vi "SDA - Analise e calibracao - backup 04.12.18.vi"() -> ()   [LabVIEW 2014]
uses:
  <vilib>/Utility/file.llb/Read From Spreadsheet File (DBL).vi
  <vilib>/Analysis/NI_AALPro.lvlib
  <vilib>/gmath/NI_Gmath.lvlib
  <vilib>/measure/NI_MABase.lvlib
panel:
  in  "Amplitude base":dbl=1.25 format="%#_13g"
  in  "p.u. ?":bool=TRUE
  in  "Numeric":dbl
  out "output cluster":cluster{i32, i32}
  in  "offset":dbl format="%0.2p"
  in  "phase":dbl format="%.2p"
  in  "amplitude":dbl=1.0 format="%0.2p"
  in  "frequency":dbl=10.0 format="%0.2p"
  out "delay time":dbl format="%#_6f"
  in  "y":dbl
  out "fractional index or x":dbl format="%#_7g"
  in  "threshold y":dbl=0.95
  out "spread value":dbl
  out "lenght":i32
  in  "kept interval":i32=25
  out "Table 2":string[][](table)
  in  "Labels Size":u32=24
  in  "X label":T1(ring)=enum."medidas"
  in  "Tab Control":T2(tab)
  in  "Tab Control 2":T3(tab)
  out "Magnitude absolute deviation":dbl[](graph)
  out "Absolute phase deviation":dbl[](graph)
  out "Magnitude deviation":dbl[](graph)
  out "Phase deviation":dbl[](graph)
  out "Phase":dbl[][](graph)
  out "Magnitude":dbl[][](graph)
  out "TVE":dbl[](graph)
  in  "Tab Control 3":T3(tab)
  out "Absolute freq. deviation":dbl[](graph)
  out "Absolute ROCOF deviation":dbl[](graph)
  out "Frequency deviation":dbl[](graph)
  out "ROCOF deviation":dbl[](graph)
  out "Frequency":dbl[][](graph)
  out "ROCOF":dbl[][](graph)
  out "Curve fit":dbl[][](graph)
  out "ROCOF\nreference":dbl[](array[numeric])
  out "ROCOF\nmeasured":dbl[](array[numeric])
  out "Frequency\nmeasured":dbl[](array[numeric])
  out "Frequency\nreference":dbl[](array[numeric])
  out "Phase\nmeasured":dbl[](array[numeric])
  out "Phase\nreference":dbl[](array[numeric])
  out "Magnitude\nmeasured":dbl[](array[numeric])
  out "Magnitude\nreference":dbl[](array[numeric])
  in  "polynomial order":i32=2
  in  "Type":T4(ring)=enum."Linear"
  out "Coefficients":string[][](table) caption="Table"
  in  "X data":T5(ring)
  in  "Y data":T5(ring)=enum."Magnitude deviation"
  out "Fit deviation":dbl[](graph)
  out "Correlation\ncoefficient (R)":dbl format="%.7g"
  out "R^2":dbl format="%.7g"
  in  "busca freq":dbl
  out "XY Graph 3":cluster{dbl[], dbl[]}(graph)
  out "XY Graph 2":cluster{dbl[], dbl[]}(graph)
  out "fractional index":dbl format="%_6g"
  out "x*y":dbl
  in  "fractional index or x 3":dbl
  out "ângulo corresp":dbl
  out "mag correspondente":dbl
  in  "frequency 2":dbl
  out "TVE Histogram":T6(graph)
  out "Frequency Error Histogram":T6(graph)
  out "Magnitude Error Histogram":T6(graph)
  out "Phase Error Histogram":T6(graph)
  in  "final":i32
  in  "Interval":bool
  in  "index":i32
  out "nº de amostras":i32
  in  "del interval":i32=25
  in  "Exclude\ninterval":bool
  in  "Archive name":path=path "D:/Resultados/teste.txt"
  # "Fase x freq"
  # "Mag. x mag."
  # "Synchrophasors Data Analysis"
  # "Main Errors"
  # "Max"
  # "Mean"
  # "Min"
  # "Magnitude (%)"
  # "Phase (º)"
  # "TVE (%)"
  # "Freq. (Hz)"
  # "ROCOF (Hz/s)"
  # "Tamanho para dissertação:\n312x732"
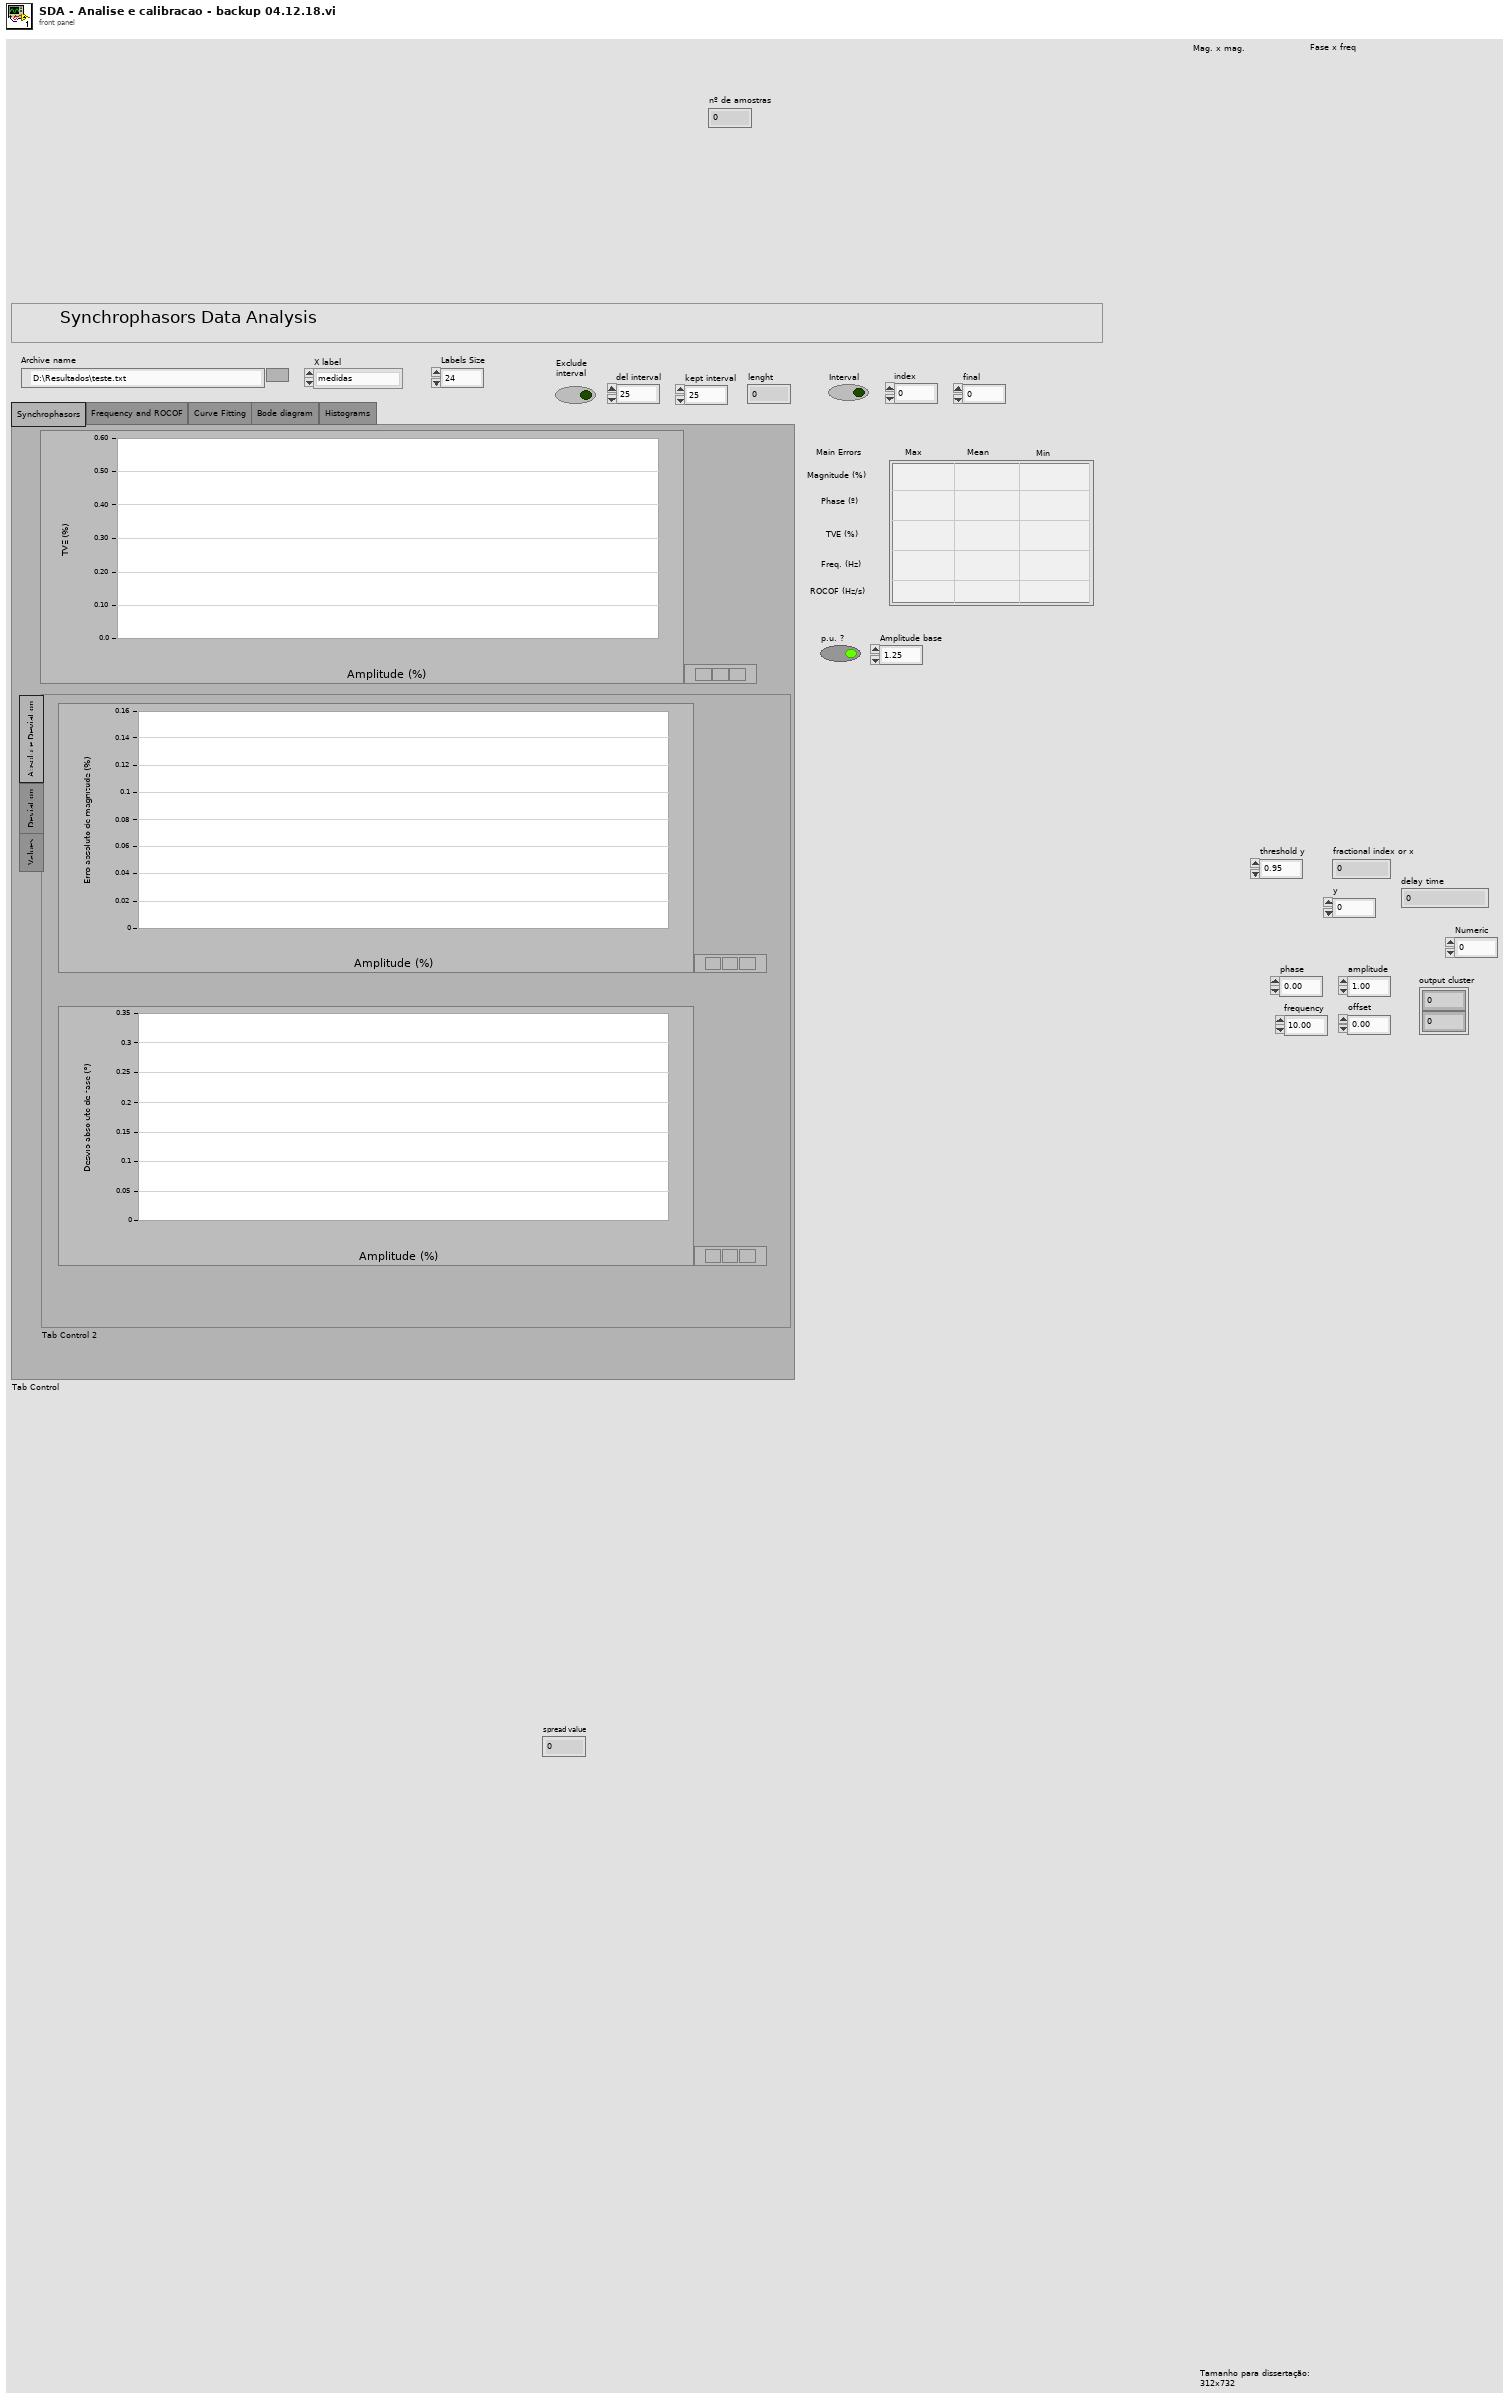
[diagram p1: front panel]
types:
  T1 = enum16{"tempo (s)", "medidas", "Amplitude (%)", "Ângulo (°)", "Frequência (Hz)", "ROCOF (Hz/s)", "Harmônica (.ª)", "Frequência de interferência (Hz)", "Frequência de modulação (Hz)"}
  T2 = enum32{"Synchrophasors", "Frequency and ROCOF", "Curve Fitting", "Bode diagram", "Histograms"}
  T3 = enum32{"Absolute Deviation", "Deviation", "Values"}
  T4 = enum16{"Exponencial", "Logarithm", "Linear", "Polynomial", "Sinusoidal"}
  T5 = enum16{"Magnitude reference", "Magnitude measured", "Magnitude deviation", "Phase reference", "Phase measured", "Phase deviation", "Frequency reference", "Frequency measured", "Frequency deviation"}
  T6 = cluster{"X Values":dbl[], "Histogram: h(x)":i32[]}
  T7 = cluster{"max ref":dbl, "min ref":dbl, "mean ref":dbl, "max dev":dbl, "min dev":dbl, "mean dev":dbl, "max meas":dbl, "min meas":dbl, "mean meas":dbl}
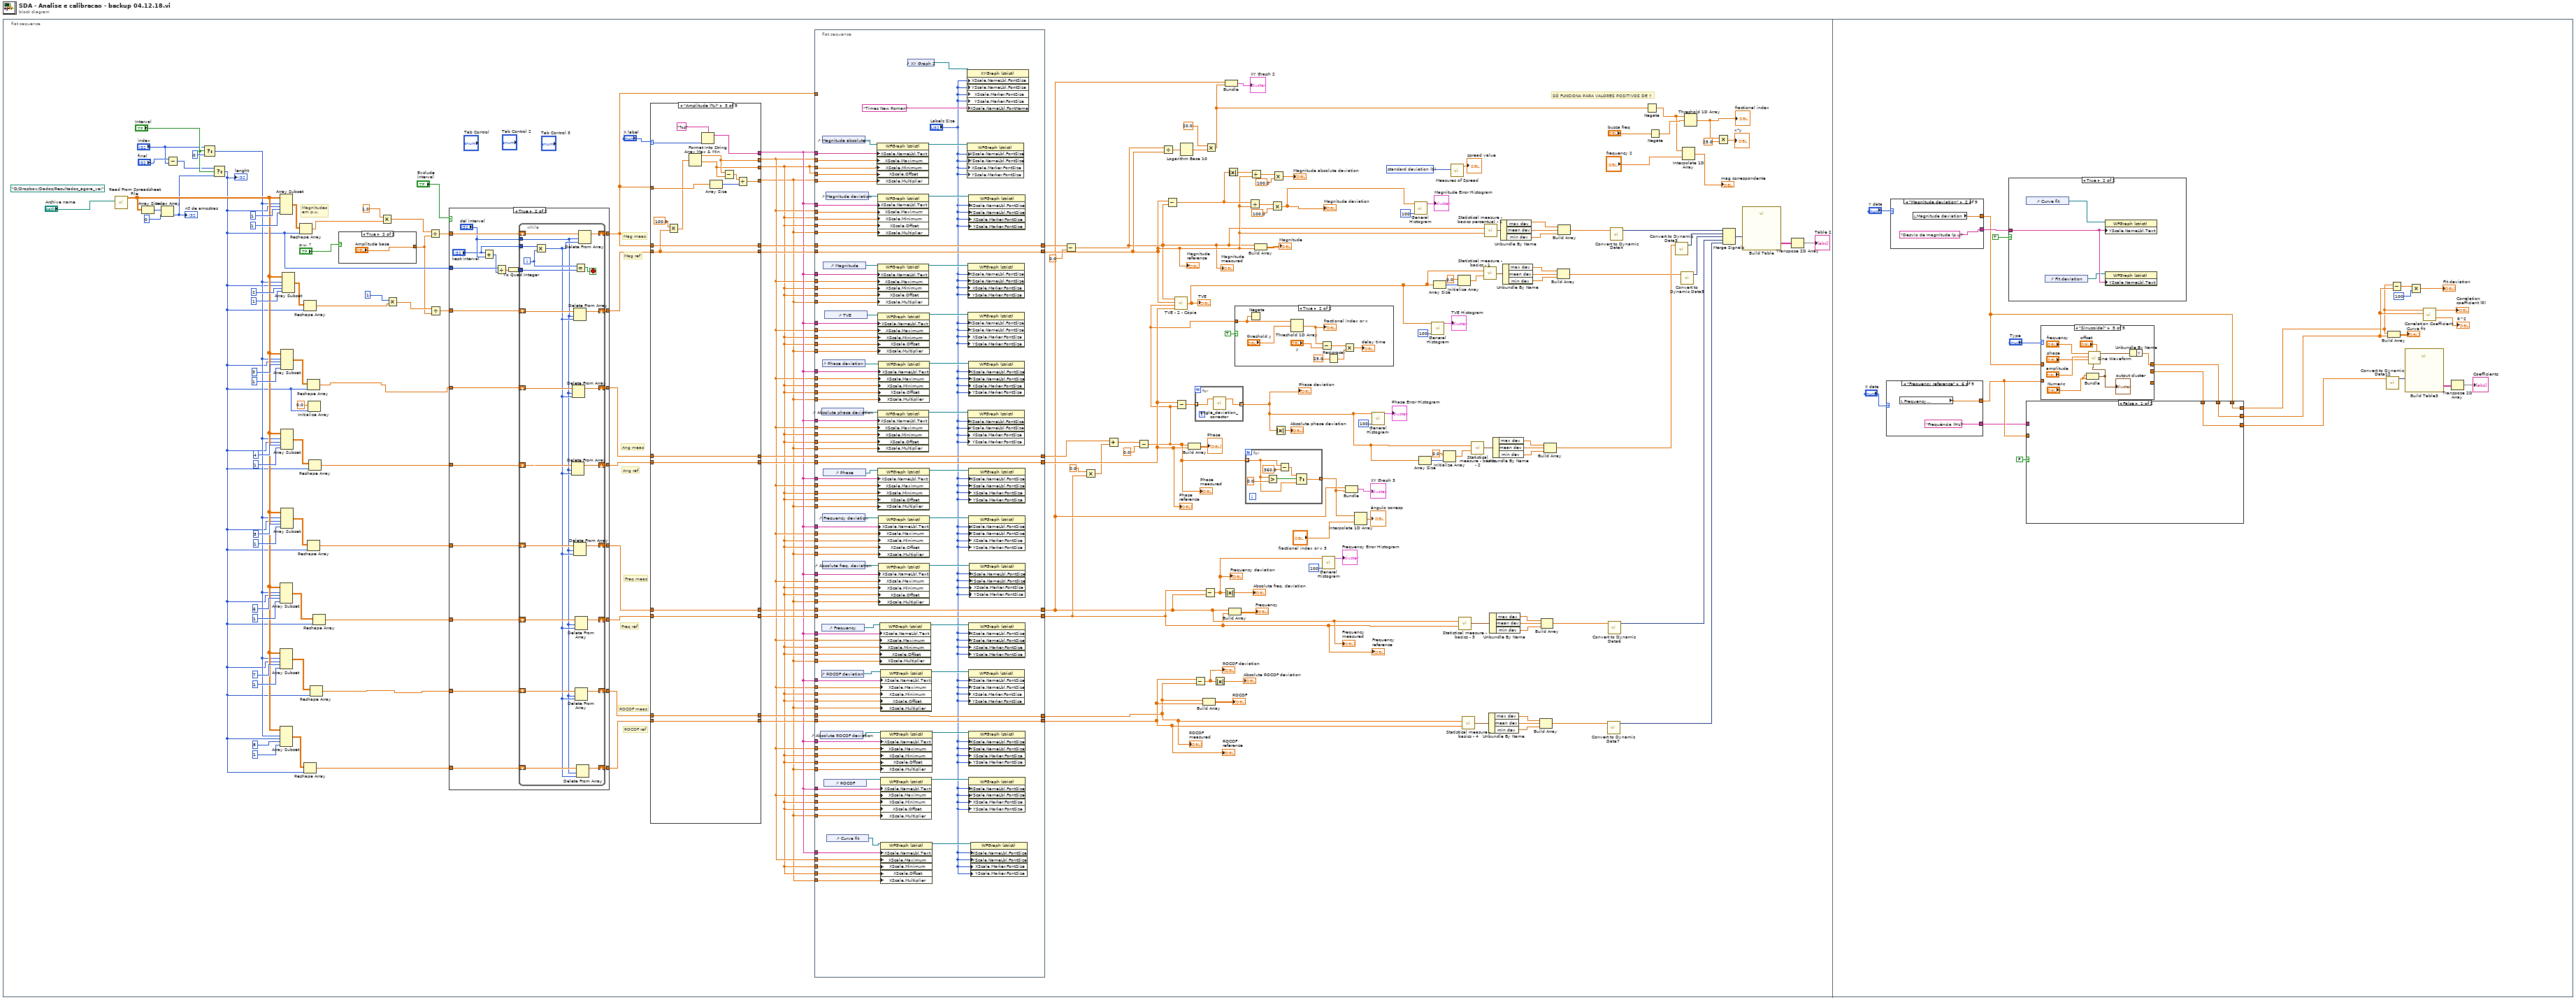
[diagram p0: block diagram]
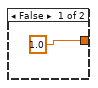
[diagram p3: hidden frame]
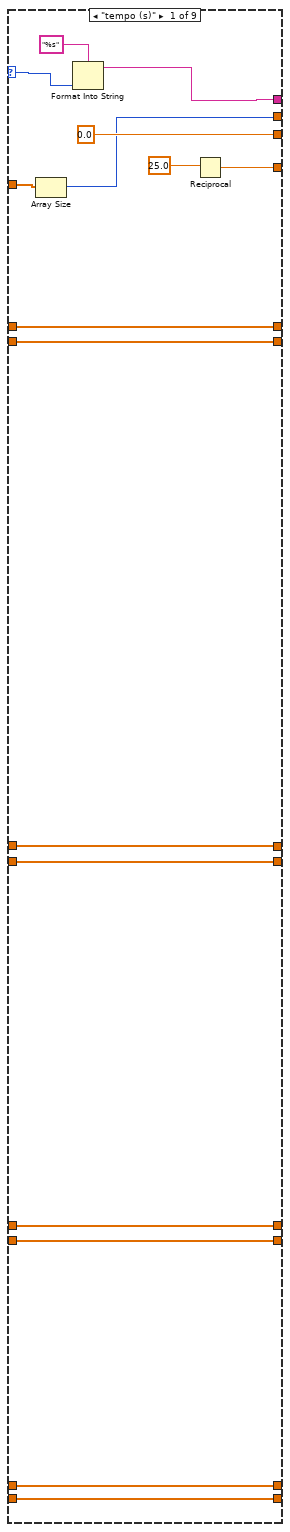
[diagram p4: hidden frame]
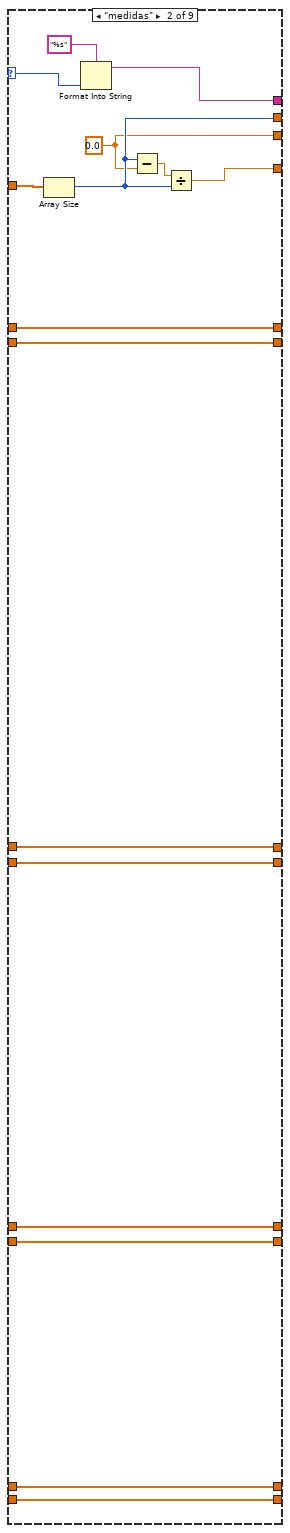
[diagram p5: hidden frame]
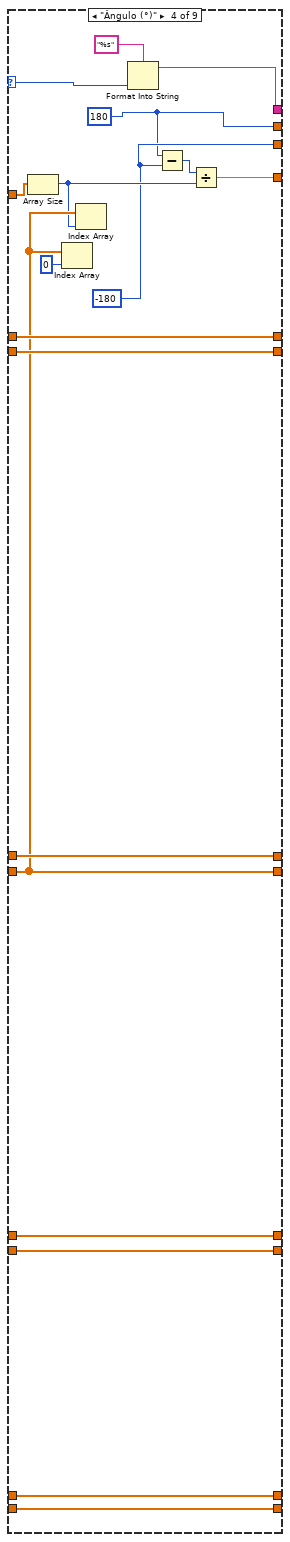
[diagram p6: hidden frame]
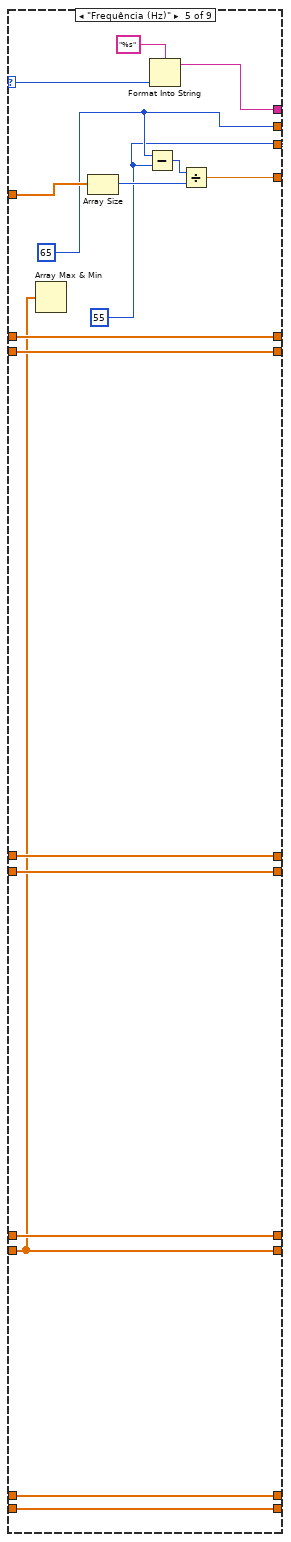
[diagram p7: hidden frame]
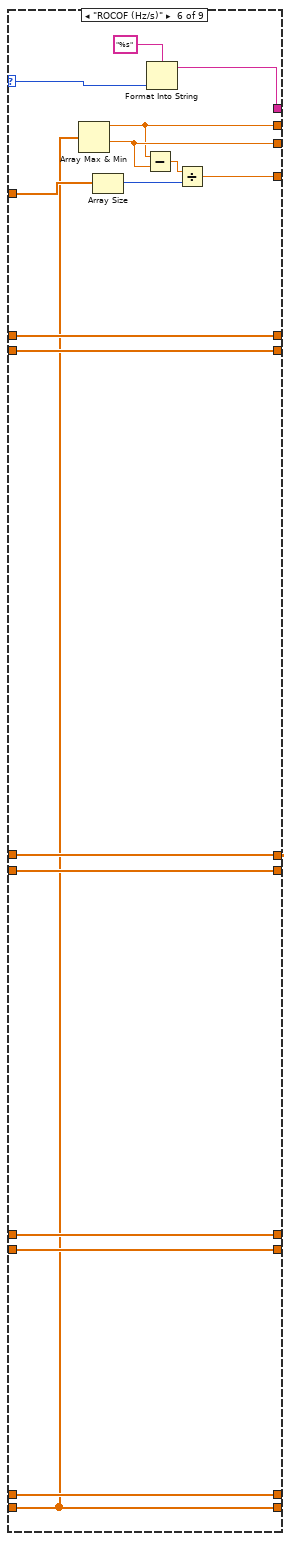
[diagram p8: hidden frame]
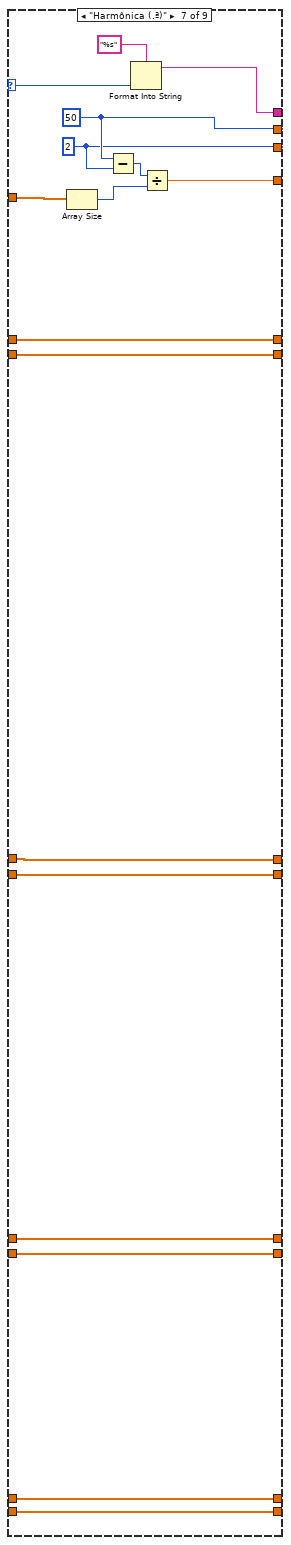
[diagram p9: hidden frame]
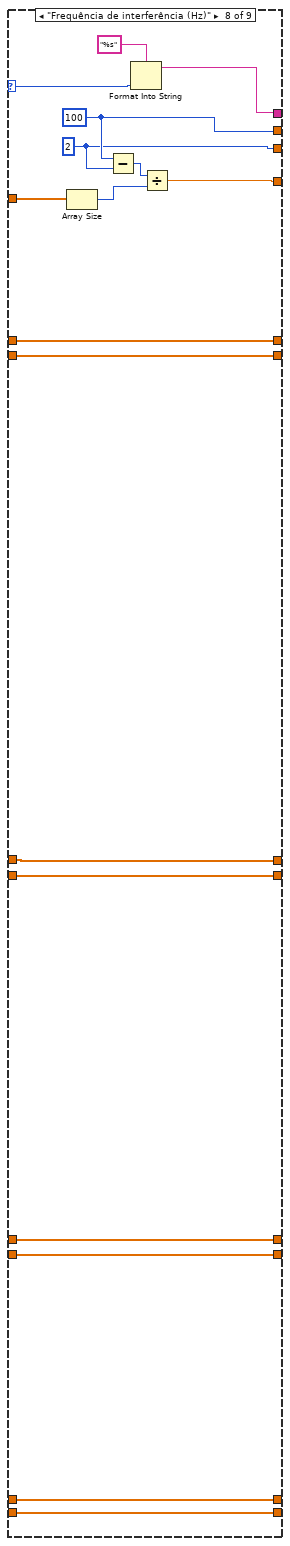
[diagram p10: hidden frame]
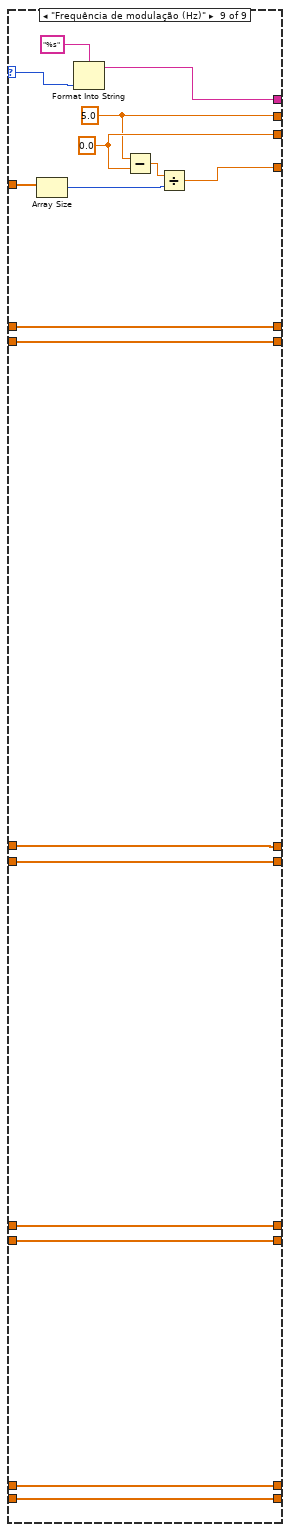
[diagram p11: hidden frame]
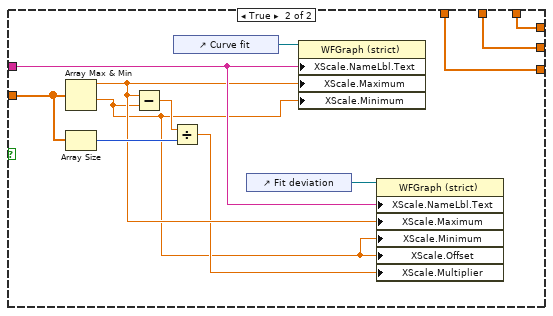
[diagram p13: hidden frame]
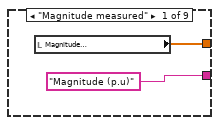
[diagram p15: hidden frame]
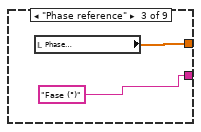
[diagram p16: hidden frame]
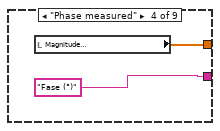
[diagram p17: hidden frame]
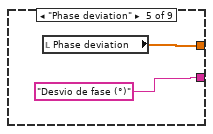
[diagram p18: hidden frame]
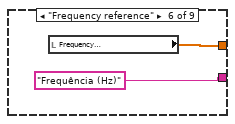
[diagram p19: hidden frame]
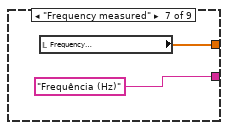
[diagram p20: hidden frame]
diagram:
  n1 = flat-sequence {
    frame #0 {
      w60 = 0 items=["standard deviation", "range", "mean absolute deviation", "interquartile range"] ("type")
      (unwired) path "D:/Dropbox/Dados/Resultados_agora_vai" ("file path (use dialog)")
      # "SÓ FUNCIONA PARA VALORES POSITIVOS DE Y"
      # "Magnitudes\nem p.u."
      # "ROCOF ref"
      # "ROCOF meas"
      # "Freq ref"
      # "Freq meas"
      # "Ang ref"
      # "Ang meas"
      # "Mag meas"
      # "Mag ref"
      n2 = call-poly <vilib>:"Read From Spreadsheet File.vi"("file path (dialog if empty)"="Archive name") -> ("all rows"=w151:dbl[][])  [unwired: 6 in, 4 out]
      n3 = Array Size(array=w151) -> (size(s)=w174:i32[])
      n4 = Index Array(array=w174, index=0) -> (element=w104:i32)
      "nº de amostras" <- w104
      n5 = Subtract(x="final", y="index") -> (x-y=w107:i32)
      n6 = Select(t="index", s="Interval", f=0) -> (s? t:f=w124:i32)
      n7 = Select(t=w107, s="Interval", f=w104) -> (s? t:f=w22:i32)
      "lenght" <- w22
      n8 = Array Subset(array=w151, index (row)=w124, length (row)=w22, index (col)=1 ("index"), length (col)=1 ("length")) -> (w175:dbl[][])
      n9 = Array Subset(array=w151, index (row)=w124, length (row)=w22, index (col)=6 ("index"), length (col)=1 ("length")) -> (w158:dbl[][])
      n10 = Array Subset(array=w151, index (row)=w124, length (row)=w22, index (col)=7 ("index"), length (col)=1 ("length")) -> (w155:dbl[][])
      n11 = Array Subset(array=w151, index (row)=w124, length (row)=w22, index (col)=8 ("index"), length (col)=1 ("length")) -> (w74:dbl[][])
      n12 = Array Subset(array=w151, index (row)=w124, length (row)=w22, index (col)=4 ("index"), length (col)=1 ("length")) -> (w164:dbl[][])
      n13 = Array Subset(array=w151, index (row)=w124, length (row)=w22, index (col)=5 ("index"), length (col)=1 ("length")) -> (w161:dbl[][])
      n14 = Array Subset(array=w151, index (row)=w124, length (row)=w22, index (col)=3 ("index"), length (col)=1 ("length")) -> (w167:dbl[][])
      n15 = Array Subset(array=w151, index (row)=w124, length (row)=w22, index (col)=2 ("index"), length (col)=1 ("length")) -> (w170:dbl[][])
      n16 = Reshape Array(w175, w22) -> (w52:dbl[])
      n17 = Reshape Array(w170, w22) -> (w50:dbl[])
      n18 = Reshape Array(w74, w22) -> (w73:dbl[])
      n19 = Reshape Array(w167, w22) -> (w21:dbl[])
      n20 = Reshape Array(w161, w22) -> (w126:dbl[])
      n21 = Initialize Array(0.0 ("element"), w22) -> ()  [unwired: 1 out]
      n22 = Reshape Array(w164, w22) -> (w125:dbl[])
      n23 = Reshape Array(w155, w22) -> (w4:dbl[])
      n24 = Reshape Array(w158, w22) -> (w127:dbl[])
      n25 = case shown="True" "p.u. ?" {
        tunnel: [1.0 "Amplitude base"] -> w3
        frame False {
        }
        frame True {
        }
      }
      n26 = Multiply(x=1.0, y=w52) -> (x*y=w51:dbl[])
      n27 = Multiply(x=1, y=w50) -> (x*y=w49:dbl[])
      n28 = Divide(x=w51, y=w3) -> (x/y=w84:dbl[])
      n29 = Divide(x=w49, y=w3) -> (x/y=w83:dbl[])
      n30 = case shown="True" "Exclude\ninterval" {
        tunnel: w84 -> [w466 w488]
        tunnel: [w466 w487] -> w41
        tunnel: w73 -> [w459 w483]
        tunnel: w4 -> [w460 w469]
        tunnel: w127 -> [w461 w480]
        tunnel: w126 -> [w462 w478]
        tunnel: w125 -> [w463 w476]
        tunnel: w21 -> [w464 w484]
        tunnel: w83 -> [w465 w486]
        tunnel: [w465 w485] -> w102
        tunnel: [w464 w474] -> w100
        tunnel: [w463 w475] -> w101
        tunnel: [w462 w477] -> w99
        tunnel: [w461 w479] -> w98
        tunnel: [w460 w481] -> w96
        tunnel: [w459 w482] -> w97
        tunnel: w22 -> [_ w473]
        frame False {
        }
        frame True {
          n31 = Add(x="kept interval", y="del interval") -> (x+y=w471:i32)
          n32 = Divide(x=w473, y=w471) -> (x/y=w468:dbl)
          n33 = To Quad Integer(1:w468) -> (0:w467:i64)
          n34 = while {
            tunnel: "del interval" -> [w490]
            shift-right: [w508] -> w487
            shift-left: w488 -> [w509]
            shift-right: [w507] -> w485
            shift-left: w486 -> [w506]
            shift-right: [w504] -> w474
            shift-left: w484 -> [w505]
            shift-right: [w502] -> w475
            shift-left: w476 -> [w503]
            shift-right: [w500] -> w477
            shift-left: w478 -> [w501]
            shift-right: [w498] -> w479
            shift-left: w480 -> [w499]
            shift-right: [w496] -> w481
            shift-left: w469 -> [w497]
            shift-right: [w494] -> w482
            shift-left: w483 -> [w495]
            tunnel: w467 -> [w493]
            tunnel: "kept interval" -> [w489]
            i -> [w492]
            stop <- w510 stop-if-true
            n35 = Multiply(x=w489, y=w492) -> (x*y=w491:i32)
            n36 = Delete From Array(array=w503, length=w490, index=w491) -> (array with subset deleted=w502:dbl[])  [unwired: 1 out]
            n37 = Delete From Array(array=w505, length=w490, index=w491) -> (array with subset deleted=w504:dbl[])  [unwired: 1 out]
            n38 = Delete From Array(array=w506, length=w490, index=w491) -> (array with subset deleted=w507:dbl[])  [unwired: 1 out]
            n39 = Delete From Array(array=w501, length=w490, index=w491) -> (array with subset deleted=w500:dbl[])  [unwired: 1 out]
            n40 = Equal?(x=w492, y=w493) -> (x = y?=w510:bool)
            n41 = Delete From Array(array=w499, length=w490, index=w491) -> (array with subset deleted=w498:dbl[])  [unwired: 1 out]
            n42 = Delete From Array(array=w497, length=w490, index=w491) -> (array with subset deleted=w496:dbl[])  [unwired: 1 out]
            n43 = Delete From Array(array=w495, length=w490, index=w491) -> (array with subset deleted=w494:dbl[])  [unwired: 1 out]
            n44 = Delete From Array(array=w509, length=w490, index=w491) -> (array with subset deleted=w508:dbl[])  [unwired: 1 out]
          }
        }
      }
      n45 = case shown="\"Amplitude (%)\"" "X label" {
        selector: "X label" -> [w310 w325 w344 w364 w380 w398 w423 w432 w451]
        tunnel: w41 -> [w311 w326 w355 w363 w381 w399 w420 w429 w452]
        tunnel: w102 -> [w319 w335 w341 w372 w378 w396 w417 w440 w454]
        tunnel: [w319 w335 w341 w372 w378 w396 w417 w440 w454] -> w86
        tunnel: w41 -> [w320 w336 w352 w373 w390 w397 w418 w441 w455]
        tunnel: [w320 w336 w352 w373 w390 w397 w418 w441 w455] -> w85
        tunnel: w101 -> [w317 w333 w350 w360 w388 w406 w416 w439 w446]
        tunnel: w100 -> [w318 w334 w351 w371 w389 w407 w408 w425 w447]
        tunnel: [w318 w334 w351 w371 w389 w407 w408 w425 w447] -> w87
        tunnel: [w317 w333 w350 w360 w388 w406 w416 w439 w446] -> w88
        tunnel: w99 -> [w316 w332 w349 w370 w387 w405 w415 w438 w445]
        tunnel: w98 -> [w315 w331 w348 w369 w377 w404 w414 w437 w444]
        tunnel: [w316 w332 w349 w370 w387 w405 w415 w438 w445] -> w90
        tunnel: [w315 w331 w348 w369 w377 w404 w414 w437 w444] -> w89
        tunnel: w97 -> [w313 w329 w347 w367 w385 w393 w412 w435 w442]
        tunnel: [w313 w329 w347 w367 w385 w393 w412 w435 w442] -> w92
        tunnel: w96 -> [w314 w330 w346 w368 w386 w403 w413 w436 w443]
        tunnel: [w314 w330 w346 w368 w386 w403 w413 w436 w443] -> w91
        tunnel: [w309 w324 w343 w362 w379 w395 w419 w433 w456] -> w57
        tunnel: [w307 w323 w339 w356 w375 w392 w411 w428 w448] -> w56
        tunnel: [0.0 ("X Scale.Offset and Multiplier:Offset") w322 w338 w357 w374 w394 w410 w427 w449] -> w55
        tunnel: [w305 w321 w337 w358 w376 w391 w409 w426 w453] -> w54
        frame "tempo (s)" {
          n46 = Array Size(array=w311) -> (size(s)=w307:i32)
          n47 = Format Into String(format string="%s", w310) -> (resulting string=w309:string)  [unwired: 2 in, 1 out]
          n48 = Reciprocal(x=25.0 ("X Scale.Offset and Multiplier:Offset")) -> (1/x=w305:dbl)
        }
        frame "medidas" {
          w322 = 0.0 ("X Scale.Offset and Multiplier:Offset")
          n49 = Array Size(array=w326) -> (size(s)=w323:i32)
          n50 = Format Into String(format string="%s", w325) -> (resulting string=w324:string)  [unwired: 2 in, 1 out]
          n51 = Subtract(x=w323, y=w322) -> (x-y=w328:dbl)
          n52 = Divide(x=w328, y=w323) -> (x/y=w321:dbl)
        }
        frame "Amplitude (%)" {
          n53 = Multiply(x=100.0 ("y"), y=w341) -> (x*y=w340:dbl[])
          n54 = Array Max & Min(array=w340) -> (max value=w339:dbl, min value=w338:dbl)  [unwired: 2 out]
          n55 = Format Into String(format string="%s", w344) -> (resulting string=w343:string)  [unwired: 2 in, 1 out]
          n56 = Array Size(array=w355) -> (size(s)=w354:i32)
          n57 = Subtract(x=w339, y=w338) -> (x-y=w353:dbl)
          n58 = Divide(x=w353, y=w354) -> (x/y=w337:dbl)
        }
        frame "Ângulo (°)" {
          w356 = 180
          w357 = -180
          n59 = Array Size(array=w363) -> (size(s)=w359:i32)
          n60 = Index Array(array=w360, index=0) -> ()  [unwired: 1 out]
          n61 = Index Array(array=w360, index=w359) -> ()  [unwired: 1 out]
          n62 = Format Into String(format string="%s", w364) -> (resulting string=w362:string)  [unwired: 2 in, 1 out]
          n63 = Subtract(x=w356, y=w357) -> (x-y=w366:i32)
          n64 = Divide(x=w366, y=w359) -> (x/y=w358:dbl)
        }
        frame "Frequência (Hz)" {
          w374 = 55
          w375 = 65
          n65 = Array Max & Min(array=w377) -> ()  [unwired: 4 out]
          n66 = Array Size(array=w381) -> (size(s)=w384:i32)
          n67 = Subtract(x=w375, y=w374) -> (x-y=w383:i32)
          n68 = Format Into String(format string="%s", w380) -> (resulting string=w379:string)  [unwired: 2 in, 1 out]
          n69 = Divide(x=w383, y=w384) -> (x/y=w376:dbl)
        }
        frame "ROCOF (Hz/s)" {
          n70 = Array Max & Min(array=w393) -> (max value=w392:dbl, min value=w394:dbl)  [unwired: 2 out]
          n71 = Array Size(array=w399) -> (size(s)=w402:i32)
          n72 = Subtract(x=w392, y=w394) -> (x-y=w401:dbl)
          n73 = Format Into String(format string="%s", w398) -> (resulting string=w395:string)  [unwired: 2 in, 1 out]
          n74 = Divide(x=w401, y=w402) -> (x/y=w391:dbl)
        }
        frame "Harmônica (.ª)" {
          w410 = 2
          w411 = 50
          n75 = Array Size(array=w420) -> (size(s)=w422:i32)
          n76 = Subtract(x=w411, y=w410) -> (x-y=w421:i32)
          n77 = Format Into String(format string="%s", w423) -> (resulting string=w419:string)  [unwired: 2 in, 1 out]
          n78 = Divide(x=w421, y=w422) -> (x/y=w409:dbl)
        }
        frame "Frequência de interferência (Hz)" {
          w427 = 2
          w428 = 100
          n79 = Array Size(array=w429) -> (size(s)=w431:i32)
          n80 = Subtract(x=w428, y=w427) -> (x-y=w430:i32)
          n81 = Format Into String(format string="%s", w432) -> (resulting string=w433:string)  [unwired: 2 in, 1 out]
          n82 = Divide(x=w430, y=w431) -> (x/y=w426:dbl)
        }
        frame "Frequência de modulação (Hz)" {
          w448 = 5.0 ("X Scale.Offset and Multiplier:Offset")
          w449 = 0.0 ("X Scale.Offset and Multiplier:Offset")
          n83 = Array Size(array=w452) -> (size(s)=w450:i32)
          n84 = Format Into String(format string="%s", w451) -> (resulting string=w456:string)  [unwired: 2 in, 1 out]
          n85 = Subtract(x=w448, y=w449) -> (x-y=w458:dbl)
          n86 = Divide(x=w458, y=w450) -> (x/y=w453:dbl)
        }
      }
      n87 = flat-sequence {
        tunnel: w57 -> [w304]
        tunnel: w57 -> [w303]
        tunnel: w57 -> [w302]
        tunnel: w56 -> [w301]
        tunnel: w55 -> [w300]
        tunnel: w55 -> [w299]
        tunnel: w54 -> [w298]
        tunnel: w56 -> [w297]
        tunnel: w55 -> [w296]
        tunnel: w55 -> [w295]
        tunnel: w54 -> [w294]
        tunnel: w57 -> [w293]
        tunnel: w57 -> [w292]
        tunnel: w57 -> [w291]
        tunnel: w54 -> [w290]
        tunnel: w55 -> [w289]
        tunnel: w55 -> [w288]
        tunnel: w56 -> [w287]
        tunnel: w54 -> [w286]
        tunnel: w55 -> [w285]
        tunnel: w55 -> [w284]
        tunnel: w56 -> [w283]
        tunnel: w57 -> [w282]
        tunnel: w54 -> [w281]
        tunnel: w55 -> [w280]
        tunnel: w55 -> [w279]
        tunnel: w56 -> [w278]
        tunnel: w56 -> [w277]
        tunnel: w55 -> [w276]
        tunnel: w55 -> [w275]
        tunnel: w54 -> [w274]
        tunnel: w56 -> [w273]
        tunnel: w55 -> [w272]
        tunnel: w55 -> [w271]
        tunnel: w54 -> [w270]
        tunnel: w57 -> [w269]
        tunnel: w57 -> [w268]
        tunnel: w56 -> [w267]
        tunnel: w55 -> [w266]
        tunnel: w55 -> [w265]
        tunnel: w54 -> [w264]
        tunnel: w57 -> [w263]
        tunnel: w56 -> [w262]
        tunnel: w55 -> [w261]
        tunnel: w55 -> [w260]
        tunnel: w54 -> [w259]
        tunnel: w57 -> [w258]
        tunnel: w56 -> [w257]
        tunnel: w55 -> [w256]
        tunnel: w55 -> [w255]
        tunnel: w54 -> [w254]
        tunnel: w57 -> [w253]
        tunnel: w56 -> [w252]
        tunnel: w55 -> [w251]
        tunnel: w55 -> [w250]
        tunnel: w54 -> [w249]
        tunnel: w57 -> [w248]
        tunnel: w56 -> [w247]
        tunnel: w55 -> [w246]
        tunnel: w55 -> [w245]
        tunnel: w54 -> [w244]
        tunnel: w54 -> [w243]
        tunnel: w55 -> [w242]
        tunnel: w55 -> [w241]
        tunnel: w56 -> [w240]
        tunnel: w92 -> [w213]
        tunnel: [w213] -> w45
        tunnel: [w212] -> w44
        tunnel: w91 -> [w212]
        tunnel: w90 -> [w211]
        tunnel: [w211] -> w2
        tunnel: w89 -> [w210]
        tunnel: [w210] -> w1
        tunnel: w88 -> [w209]
        tunnel: w87 -> [w208]
        tunnel: [w209] -> w61
        tunnel: [w208] -> w11
        tunnel: [w206] -> w13
        tunnel: [w207] -> w43
        tunnel: w86 -> [w207]
        tunnel: w85 -> [w206]
        tunnel: w57 -> [w203]
        tunnel: w56 -> [w202]
        tunnel: w55 -> [w201]
        tunnel: w55 -> [w200]
        tunnel: w54 -> [w199]
        tunnel: w41 -> [_]
        frame #0 {
          n88 = control-ref of="Absolute ROCOF deviation"() -> (w223:refnum<vi>)
          n89 = control-ref of="Absolute phase deviation"() -> (w230:refnum<vi>)
          n90 = control-ref of="ROCOF deviation"() -> (w224:refnum<vi>)
          n91 = control-ref of="Frequency"() -> (w225:refnum<vi>)
          n92 = control-ref of="Magnitude absolute deviation"() -> (w215:refnum<vi>)
          n93 = control-ref of="Phase deviation"() -> (w231:refnum<vi>)
          n94 = control-ref of="Absolute freq. deviation"() -> (w226:refnum<vi>)
          n95 = control-ref of="Frequency deviation"() -> (w227:refnum<vi>)
          n96 = control-ref of="Magnitude"() -> (w214:refnum<vi>)
          n97 = control-ref of="Phase"() -> (w229:refnum<vi>)
          n98 = control-ref of="ROCOF"() -> (w222:refnum<vi>)
          n99 = control-ref of="TVE"() -> (w232:refnum<vi>)
          n100 = control-ref of="Magnitude deviation"() -> (w238:refnum<vi>)
          n101 = control-ref of="Curve fit"() -> (w204:refnum<vi>)
          n102 = property on="Property Node" class="WFGraph (strict)"(reference=w215, "XScale.NameLbl.Text"=w304, "XScale.Maximum"=w301, "XScale.Minimum"=w300, "XScale.Offset"=w299, "XScale.Multiplier"=w298) -> (reference out=w239:refnum<vi>)  [unwired: 1 in, 1 out]
          n103 = property on="Property Node" class="WFGraph (strict)"(reference=w238, "XScale.NameLbl.Text"=w303, "XScale.Maximum"=w297, "XScale.Minimum"=w296, "XScale.Offset"=w295, "XScale.Multiplier"=w294) -> (reference out=w237:refnum<vi>)  [unwired: 1 in, 1 out]
          n104 = property on="Property Node" class="WFGraph (strict)"(reference=w214, "XScale.NameLbl.Text"=w302, "XScale.Maximum"=w283, "XScale.Minimum"=w284, "XScale.Offset"=w285, "XScale.Multiplier"=w286) -> (reference out=w235:refnum<vi>)  [unwired: 1 in, 1 out]
          n105 = property on="Property Node" class="WFGraph (strict)"(reference=w230, "XScale.NameLbl.Text"=w293, "XScale.Maximum"=w273, "XScale.Minimum"=w272, "XScale.Offset"=w271, "XScale.Multiplier"=w270) -> (reference out=w233:refnum<vi>)  [unwired: 1 in, 1 out]
          n106 = property on="Property Node" class="WFGraph (strict)"(reference=w232, "XScale.NameLbl.Text"=w291, "XScale.Maximum"=w287, "XScale.Minimum"=w288, "XScale.Offset"=w289, "XScale.Multiplier"=w290) -> (reference out=w236:refnum<vi>)  [unwired: 1 in, 1 out]
          n107 = property on="Property Node" class="WFGraph (strict)"(reference=w229, "XScale.NameLbl.Text"=w282, "XScale.Maximum"=w278, "XScale.Minimum"=w279, "XScale.Offset"=w280, "XScale.Multiplier"=w281) -> (reference out=w228:refnum<vi>)  [unwired: 1 in, 1 out]
          n108 = property on="Property Node" class="WFGraph (strict)"(reference=w231, "XScale.NameLbl.Text"=w292, "XScale.Maximum"=w277, "XScale.Minimum"=w276, "XScale.Offset"=w275, "XScale.Multiplier"=w274) -> (reference out=w234:refnum<vi>)  [unwired: 1 in, 1 out]
          n109 = property on="Property Node" class="WFGraph (strict)"(reference=w227, "XScale.NameLbl.Text"=w269, "XScale.Maximum"=w240, "XScale.Minimum"=w241, "XScale.Offset"=w242, "XScale.Multiplier"=w243) -> (reference out=w221:refnum<vi>)  [unwired: 1 in, 1 out]
          n110 = property on="Property Node" class="WFGraph (strict)"(reference=w226, "XScale.NameLbl.Text"=w268, "XScale.Maximum"=w267, "XScale.Minimum"=w266, "XScale.Offset"=w265, "XScale.Multiplier"=w264) -> (reference out=w220:refnum<vi>)  [unwired: 1 in, 1 out]
          n111 = property on="Property Node" class="WFGraph (strict)"(reference=w225, "XScale.NameLbl.Text"=w263, "XScale.Maximum"=w262, "XScale.Minimum"=w261, "XScale.Offset"=w260, "XScale.Multiplier"=w259) -> (reference out=w219:refnum<vi>)  [unwired: 1 in, 1 out]
          n112 = property on="Property Node" class="WFGraph (strict)"(reference=w224, "XScale.NameLbl.Text"=w258, "XScale.Maximum"=w257, "XScale.Minimum"=w256, "XScale.Offset"=w255, "XScale.Multiplier"=w254) -> (reference out=w218:refnum<vi>)  [unwired: 1 in, 1 out]
          n113 = property on="Property Node" class="WFGraph (strict)"(reference=w222, "XScale.NameLbl.Text"=w248, "XScale.Maximum"=w247, "XScale.Minimum"=w246, "XScale.Offset"=w245, "XScale.Multiplier"=w244) -> (reference out=w216:refnum<vi>)  [unwired: 1 in, 1 out]
          n114 = property on="Property Node" class="WFGraph (strict)"(reference=w223, "XScale.NameLbl.Text"=w253, "XScale.Maximum"=w252, "XScale.Minimum"=w251, "XScale.Offset"=w250, "XScale.Multiplier"=w249) -> (reference out=w217:refnum<vi>)  [unwired: 1 in, 1 out]
          n115 = property on="Property Node" class="WFGraph (strict)"(reference=w204, "XScale.NameLbl.Text"=w203, "XScale.Maximum"=w202, "XScale.Minimum"=w201, "XScale.Offset"=w200, "XScale.Multiplier"=w199) -> (reference out=w205:refnum<vi>)  [unwired: 1 in, 1 out]
          n116 = control-ref of="XY Graph 2"() -> (w198:refnum<vi>)
          n117 = property class="XYGraph (strict)"(reference=w198, "XScale.NameLbl.FontSize"="Labels Size", "YScale.NameLbl.FontSize"="Labels Size", "XScale.Marker.FontSize"="Labels Size", "YScale.Marker.FontSize"="Labels Size", "XScale.NameLbl.FontName"="Times New Roman" ("X Scale.Name Label.Font:Name")) -> ()  [unwired: 1 in, 2 out]
          n118 = property class="WFGraph (strict)"(reference=w239, "XScale.NameLbl.FontSize"="Labels Size", "YScale.NameLbl.FontSize"="Labels Size", "XScale.Marker.FontSize"="Labels Size", "YScale.Marker.FontSize"="Labels Size") -> ()  [unwired: 1 in, 2 out]
          n119 = property class="WFGraph (strict)"(reference=w235, "XScale.NameLbl.FontSize"="Labels Size", "YScale.NameLbl.FontSize"="Labels Size", "XScale.Marker.FontSize"="Labels Size", "YScale.Marker.FontSize"="Labels Size") -> ()  [unwired: 1 in, 2 out]
          n120 = property class="WFGraph (strict)"(reference=w236, "XScale.NameLbl.FontSize"="Labels Size", "YScale.NameLbl.FontSize"="Labels Size", "XScale.Marker.FontSize"="Labels Size", "YScale.Marker.FontSize"="Labels Size") -> ()  [unwired: 1 in, 2 out]
          n121 = property class="WFGraph (strict)"(reference=w233, "XScale.NameLbl.FontSize"="Labels Size", "YScale.NameLbl.FontSize"="Labels Size", "XScale.Marker.FontSize"="Labels Size", "YScale.Marker.FontSize"="Labels Size") -> ()  [unwired: 1 in, 2 out]
          n122 = property class="WFGraph (strict)"(reference=w234, "XScale.NameLbl.FontSize"="Labels Size", "YScale.NameLbl.FontSize"="Labels Size", "XScale.Marker.FontSize"="Labels Size", "YScale.Marker.FontSize"="Labels Size") -> ()  [unwired: 1 in, 2 out]
          n123 = property class="WFGraph (strict)"(reference=w218, "XScale.NameLbl.FontSize"="Labels Size", "YScale.NameLbl.FontSize"="Labels Size", "XScale.Marker.FontSize"="Labels Size", "YScale.Marker.FontSize"="Labels Size") -> ()  [unwired: 1 in, 2 out]
          n124 = property class="WFGraph (strict)"(reference=w237, "XScale.NameLbl.FontSize"="Labels Size", "YScale.NameLbl.FontSize"="Labels Size", "XScale.Marker.FontSize"="Labels Size", "YScale.Marker.FontSize"="Labels Size") -> ()  [unwired: 1 in, 2 out]
          n125 = property class="WFGraph (strict)"(reference=w228, "XScale.NameLbl.FontSize"="Labels Size", "YScale.NameLbl.FontSize"="Labels Size", "XScale.Marker.FontSize"="Labels Size", "YScale.Marker.FontSize"="Labels Size") -> ()  [unwired: 1 in, 2 out]
          n126 = property class="WFGraph (strict)"(reference=w221, "XScale.NameLbl.FontSize"="Labels Size", "YScale.NameLbl.FontSize"="Labels Size", "XScale.Marker.FontSize"="Labels Size", "YScale.Marker.FontSize"="Labels Size") -> ()  [unwired: 1 in, 2 out]
          n127 = property class="WFGraph (strict)"(reference=w219, "XScale.NameLbl.FontSize"="Labels Size", "YScale.NameLbl.FontSize"="Labels Size", "XScale.Marker.FontSize"="Labels Size", "YScale.Marker.FontSize"="Labels Size") -> ()  [unwired: 1 in, 2 out]
          n128 = property class="WFGraph (strict)"(reference=w217, "XScale.NameLbl.FontSize"="Labels Size", "YScale.NameLbl.FontSize"="Labels Size", "XScale.Marker.FontSize"="Labels Size", "YScale.Marker.FontSize"="Labels Size") -> ()  [unwired: 1 in, 2 out]
          n129 = property class="WFGraph (strict)"(reference=w216, "XScale.NameLbl.FontSize"="Labels Size", "YScale.NameLbl.FontSize"="Labels Size", "XScale.Marker.FontSize"="Labels Size", "YScale.Marker.FontSize"="Labels Size") -> ()  [unwired: 1 in, 2 out]
          n130 = property class="WFGraph (strict)"(reference=w220, "XScale.NameLbl.FontSize"="Labels Size", "YScale.NameLbl.FontSize"="Labels Size", "XScale.Marker.FontSize"="Labels Size", "YScale.Marker.FontSize"="Labels Size") -> ()  [unwired: 1 in, 2 out]
          n131 = property class="WFGraph (strict)"(reference=w205, "XScale.NameLbl.FontSize"="Labels Size", "YScale.NameLbl.FontSize"="Labels Size", "XScale.Marker.FontSize"="Labels Size", "YScale.Marker.FontSize"="Labels Size") -> ()  [unwired: 1 in, 2 out]
        }
      }
      n132 = Subtract(x=w13, y=0.0 ("x")) -> (x-y=w12:dbl[])
      "Magnitude\nmeasured" <- w12
      n133 = Multiply(x=0.0, y=w1) -> (x*y=w10:dbl[])
      n134 = Add(x=w11, y=w10) -> (x+y=w7:dbl[])
      n135 = Subtract(x=w7, y=0.0 ("x")) -> (x-y=w8:dbl[])
      "Phase\nmeasured" <- w8
      n136 = Divide(x=w12, y=w43) -> (x/y=w38:dbl[])
      n137 = Subtract(x=w43, y=w12) -> (x-y=w111:dbl[])
      n138 = call "TVE - 2 - Cópia.vi"("Angle reference"=w61, "Angle measured"=w8, "Voltage reference"=w43, "Voltage measured"=w12) -> ("Array"=w20:dbl[])
      "TVE" <- w20
      n139 = Subtract(x=w61, y=w8) -> (x-y=w157:dbl[])
      n140 = Logarithm Base 10(1:w38) -> (0:w42:dbl[])
      n141 = Build Array(w8, w61) -> (→"Phase":dbl[][])
      n142 = Subtract(x=w45, y=w44) -> (x-y=w108:dbl[])
      "ROCOF deviation" <- w108
      n143 = for {
        tunnel: w157 -> [w194] mode=indexing
        tunnel: [w195] -> w16 mode=indexing
        n144 = call "angle_deviation_corrector.vi"("angle"=w194) -> ("angle corrected"=w195:dbl)  [unwired: 6 in, 2 out]
      }
      "Phase deviation" <- w16
      n145 = Build Array(w44, w45) -> (→"ROCOF":dbl[][])
      n146 = Subtract(x=w1, y=w2) -> (x-y=w19:dbl[])
      "Frequency deviation" <- w19
      n147 = Multiply(x=20.0, y=w42) -> (x*y=w32:dbl[])
      n148 = Absolute Value(x=w108) -> (abs(x)=→"Absolute ROCOF deviation":dbl[])
      n149 = Absolute Value(x=w19) -> (abs(x)=→"Absolute freq. deviation":dbl[])
      n150 = Bundle(w2, w32) -> (→"XY Graph 2":cluster{dbl[], dbl[]})  [unwired: 1 in]
      n151 = Absolute Value(x=w111) -> (abs(x)=w115:dbl[])
      n152 = Build Array(w2, w1) -> (→"Frequency":dbl[][])
      n153 = case shown="True" TRUE {
        tunnel: w8 -> [_ w178]
        frame False {
        }
        frame True {
          n154 = Negate(x=w178) -> ()  [unwired: 1 out]
          n155 = Threshold 1D Array(2:"threshold y", 3:w178) -> (0:w185:dbl)  [unwired: 1 in]
          "fractional index or x" <- w185
          n156 = Subtract(x=w185, y="y") -> (x-y=w184:dbl)
          n157 = Reciprocal(x=25.0) -> (1/x=w182:dbl)
          n158 = Multiply(x=w184, y=w182) -> (x*y=→"delay time":dbl)
        }
      }
      n159 = for {
        tunnel: w8 -> [w188] mode=indexing
        tunnel: [w186] -> w29 mode=indexing
        n160 = Greater?(x=w188, y=0.0) -> (0:w190:bool)
        n161 = Subtract(x=w188, y=360.0) -> (x-y=w187:dbl)
        n162 = Select(t=w187, s=w190, f=w188) -> (s? t:f=w186:dbl)
      }
      n163 = Divide(x=w111, y=w43) -> (x/y=w113:dbl[])
      n164 = Divide(x=w115, y=w43) -> (x/y=w116:dbl[])
      n165 = Build Array(w12, w43) -> (→"Magnitude":dbl[][])
      n166 = Multiply(x=w113, y=100.0 ("x")) -> (x*y=w15:dbl[])
      "Magnitude deviation" <- w15
      n167 = Multiply(x=w116, y=100.0 ("x")) -> (x*y=→"Magnitude absolute deviation":dbl[])
      n168 = Absolute Value(x=w16) -> (abs(x)=→"Absolute phase deviation":dbl[])
      n169 = call <vilib>:"General Histogram.vi"("X"=w19, "# bins"=100) -> ("Histogram Graph"=→"Frequency Error Histogram":T6)  [unwired: 9 in, 4 out]
      n170 = Bundle(w2, w29) -> (→"XY Graph 3":cluster{dbl[], dbl[]})  [unwired: 1 in]
      n171 = Interpolate 1D Array(1:"fractional index or x 3", 2:w29) -> (0:→"ângulo corresp":dbl)
      n172 = call <vilib>:"General Histogram.vi"("X"=w16, "# bins"=100) -> ("Histogram Graph"=→"Phase Error Histogram":T6)  [unwired: 9 in, 4 out]
      n173 = call <vilib>:"General Histogram.vi"("X"=w15, "# bins"=100) -> ("Histogram Graph"=→"Magnitude Error Histogram":T6)  [unwired: 9 in, 4 out]
      n174 = Array Size(array=w16) -> (size(s)=w120:i32)
      n175 = call <vilib>:"General Histogram.vi"("X"=w20, "# bins"=100) -> ("Histogram Graph"=→"TVE Histogram":T6)  [unwired: 9 in, 4 out]
      n176 = Array Size(array=w20) -> (size(s)=w147:i32)
      n177 = Initialize Array(0.0 ("element"), w120) -> (w118:dbl[])
      n178 = call <vilib>:"Measures of Spread.vi"("type"=w60) -> ("spread value"=→"spread value":dbl)  [unwired: 9 in, 1 out]
      n179 = Initialize Array(0.0 ("element"), w147) -> (w145:dbl[])
      n180 = call "Statistical measure - basics - 3.vi"("Data measured"=w2, "Data reference"=w1) -> ("Statistcs"=w137:T7)  [unwired: 12 in, 1 out]
      n181 = call "Statistical measure - basics - 4.vi"("Data measured"=w44, "Data reference"=w45) -> ("Statistcs"=w134:T7)  [unwired: 12 in, 1 out]
      n182 = call "Statistical measure - basics - 2.vi"("Data measured"=w16, "Data reference"=w118) -> ("Statistcs"=w141:T7)  [unwired: 12 in, 1 out]
      n183 = call "Statistical measure - basics - 1.vi"("Data measured"=w20, "Data reference"=w145) -> ("Statistcs"=w144:T7)  [unwired: 12 in, 1 out]
      n184 = call "Statistical measure - basics percentual - 1.vi"("Data measured"=w12, "Data reference"=w43) -> ("Statistcs"=w150:T7)  [unwired: 12 in, 1 out]
      n185 = Unbundle By Name(w134) -> ("max dev"=w78:dbl, "mean dev"=w136:dbl, "min dev"=w135:dbl)
      n186 = Unbundle By Name(w137) -> ("max dev"=w79:dbl, "mean dev"=w138:dbl, "min dev"=w121:dbl)
      n187 = Unbundle By Name(w141) -> ("max dev"=w80:dbl, "mean dev"=w140:dbl, "min dev"=w139:dbl)
      n188 = Unbundle By Name(w150) -> ("max dev"=w82:dbl, "mean dev"=w149:dbl, "min dev"=w148:dbl)
      n189 = Unbundle By Name(w144) -> ("max dev"=w81:dbl, "mean dev"=w143:dbl, "min dev"=w142:dbl)
      n190 = Build Array(w78, w136, w135) -> (w75:dbl[])
      n191 = Build Array(w79, w138, w121) -> (w76:dbl[])
      n192 = Build Array(w80, w140, w139) -> (w72:dbl[])
      n193 = Build Array(w81, w143, w142) -> (w71:dbl[])
      n194 = Build Array(w82, w149, w148) -> (w77:dbl[])
      n195 = call "Convert to Dynamic Data7"("Array"=w75) -> ("Dynamic Data Type"=w129:dynamicdata)  [unwired: 3 in]
      n196 = call "Convert to Dynamic Data6"("Array"=w76) -> ("Dynamic Data Type"=w130:dynamicdata)  [unwired: 3 in]
      n197 = call "Convert to Dynamic Data4"("Array"=w77) -> ("Dynamic Data Type"=w133:dynamicdata)  [unwired: 3 in]
      n198 = Negate(x=w32) -> (-x=w26:dbl[])
      n199 = Negate(x="busca freq") -> (-x=w30:dbl)
      n200 = call "Convert to Dynamic Data3"("Array"=w72) -> ("Dynamic Data Type"=w132:dynamicdata)  [unwired: 3 in]
      n201 = call "Convert to Dynamic Data5"("Array"=w71) -> ("Dynamic Data Type"=w131:dynamicdata)  [unwired: 3 in]
      n202 = Interpolate 1D Array(1:"frequency 2", 2:w26) -> (0:→"mag correspondente":dbl)
      n203 = Threshold 1D Array(2:w30, 3:w26) -> (0:w35:dbl)  [unwired: 1 in]
      "fractional index" <- w35
      n204 = Multiply(x=w35, y=25.0) -> (x*y=→"x*y":dbl)
      n205 = Merge Signals(w133, w132, w131, w130, w129) -> (w128:dynamicdata)
      n206 = call "Build Table"("Signals"=w128) -> ("Table"=w94:string[][])  [unwired: 4 in, 6 out]
      n207 = Transpose 2D Array(2D array=w94) -> (transposed array=→"Table 2":string[][])
      "ROCOF\nreference" <- w45
      "ROCOF\nmeasured" <- w44
      "Frequency\nreference" <- w1
      "Frequency\nmeasured" <- w2
      "Phase\nreference" <- w61
      "Magnitude\nreference" <- w43
    }
    frame #1 {
      n208 = case shown="\"Frequency reference\"" "X data" {
        tunnel: [w571 w573 w575 w577 w579 w581 w583 w585 w587] -> w527
        tunnel: ["Magnitude (p.u)" "Desvio de magnitude (p.u)" "Fase (°)" "Fase (°)" "Desvio de fase (°)" "Frequência (Hz)" "Frequência (Hz)" "Desvio de frequência (Hz)" "Magnitude (p.u)"] -> w526
        frame "Magnitude measured" {
          n209 = local read "Magnitude\nmeasured"() -> (w571:dbl[])
        }
        frame "Magnitude deviation" {
          n210 = local read "Magnitude deviation"() -> (w573:dbl[])
        }
        frame "Phase reference" {
          n211 = local read "Phase\nreference"() -> (w575:dbl[])
        }
        frame "Phase measured" {
          n212 = local read "Phase\nmeasured"() -> (w577:dbl[])
        }
        frame "Phase deviation" {
          n213 = local read "Phase deviation"() -> (w579:dbl[])
        }
        frame "Frequency reference" {
          n214 = local read "Frequency\nreference"() -> (w581:dbl[])
        }
        frame "Frequency measured" {
          n215 = local read "Frequency\nmeasured"() -> (w583:dbl[])
        }
        frame "Frequency deviation" {
          n216 = local read "Frequency deviation"() -> (w585:dbl[])
        }
        frame "Magnitude reference" {
          n217 = local read "Magnitude\nreference"() -> (w587:dbl[])
        }
      }
      n218 = case shown="\"Magnitude deviation\"" "Y data" {
        tunnel: [w553 w555 w557 w559 w561 w563 w565 w567 w569] -> w520
        tunnel: ["Magnitude (p.u)" "Desvio de magnitude (p.u)" "Fase (°)" "Fase (°)" "Desvio de fase (°)" "Frequência (Hz)" "Frequência (Hz)" "Desvio de frequência (Hz)" "Magnitude (p.u)"] -> w525
        frame "Magnitude measured" {
          n219 = local read "Magnitude\nmeasured"() -> (w553:dbl[])
        }
        frame "Magnitude deviation" {
          n220 = local read "Magnitude deviation"() -> (w555:dbl[])
        }
        frame "Phase reference" {
          n221 = local read "Phase\nreference"() -> (w557:dbl[])
        }
        frame "Phase measured" {
          n222 = local read "Magnitude\nmeasured"() -> (w559:dbl[])
        }
        frame "Phase deviation" {
          n223 = local read "Phase deviation"() -> (w561:dbl[])
        }
        frame "Frequency reference" {
          n224 = local read "Frequency\nreference"() -> (w563:dbl[])
        }
        frame "Frequency measured" {
          n225 = local read "Frequency\nmeasured"() -> (w565:dbl[])
        }
        frame "Frequency deviation" {
          n226 = local read "Frequency deviation"() -> (w567:dbl[])
        }
        frame "Magnitude reference" {
          n227 = local read "Magnitude\nreference"() -> (w569:dbl[])
        }
      }
      n228 = case shown="True" TRUE {
        tunnel: w525 -> [_ w551]
        frame False {
        }
        frame True {
          n229 = control-ref of="Curve fit"() -> (w550:refnum<vi>)
          n230 = control-ref of="Fit deviation"() -> (w549:refnum<vi>)
          n231 = property on="Property Node" class="WFGraph (strict)"(reference=w550, "YScale.NameLbl.Text"=w551) -> ()  [unwired: 1 in, 2 out]
          n232 = property on="Property Node" class="WFGraph (strict)"(reference=w549, "YScale.NameLbl.Text"=w551) -> ()  [unwired: 1 in, 2 out]
        }
      }
      n233 = case shown="\"Sinusoidal\"" "Type" {
        tunnel: w520 -> [w594 w602 w610 w616 _]
        tunnel: w527 -> [w593 w601 w609 w615 _]
        tunnel: [w589 w595 w605 w614 _] -> w522
        tunnel: [w592 w599 w604 w613 w623] -> w521
        tunnel: [w588 w600 w608 w612 _] -> _
        frame "Linear" {
          n234 = call <vilib>:"Linear Fit.vi"("Y"=w594, "X"=w593) -> ("Best Linear Fit"=w592:dbl[], "slope"=w591:dbl, "intercept"=w590:dbl, "residue"=w588:dbl)  [unwired: 9 in, 1 out]
          n235 = Build Array(w591, w590) -> (w589:dbl[])
        }
        frame "Exponencial" {
          n236 = call <vilib>:"Exponential Fit.vi"("Y"=w602, "X"=w601) -> ("Best Exponential Fit"=w599:dbl[], "amplitude"=w598:dbl, "damping"=w597:dbl, "offset"=w596:dbl, "residue"=w600:dbl)  [unwired: 8 in, 1 out]
          n237 = Build Array(w598, w597, w596) -> (w595:dbl[])
        }
        frame "Logarithm" {
          w603 = 2.71828 items=["e"=2.71828, "2"=2.0, "10"=10.0] ("base")
          n238 = call <vilib>:"Logarithm Fit.vi"("Y"=w610, "base"=w603, "X"=w609) -> ("Best Logarithm Fit"=w604:dbl[], "amplitude"=w607:dbl, "scale"=w606:dbl, "residue"=w608:dbl)  [unwired: 8 in, 1 out]
          n239 = Build Array(w607, w606) -> (w605:dbl[])
        }
        frame "Polynomial" {
          n240 = call <vilib>:"General Polynomial Fit.vi"("Y"=w616, "polynomial order"="polynomial order", "X"=w615) -> ("Best Polynomial Fit"=w613:dbl[], "Polynomial Coefficients"=w614:dbl[], "residue"=w612:dbl)  [unwired: 9 in, 1 out]
        }
        frame "Sinusoidal" {
          n241 = Bundle("Numeric"="Numeric", "Numeric"="Numeric") -> (w618:cluster{"Numeric":dbl, "Numeric":dbl})  [unwired: 1 in]
          "output cluster" <- w618
          n242 = call <vilib>:"Sine Waveform.vi"("offset"="offset", "sampling info"=w618, "phase"="phase", "amplitude"="amplitude", "frequency"="frequency") -> ("signal out"=w624:waveform(dbl))  [unwired: 5 in, 1 out]
          n243 = Unbundle By Name(w624) -> ("Y"=w623:dbl[])
        }
      }
      n244 = case shown="False" FALSE {
        tunnel: w527 -> [_ w548]
        tunnel: w526 -> [_ w547]
        tunnel: w522 -> [w534 w537]
        tunnel: w521 -> [w535 w538]
        tunnel: w520 -> [w536 w539]
        tunnel: [w536 w539] -> w531
        tunnel: [w535 w538] -> w532
        tunnel: [w534 w537] -> w533
        frame False {
        }
        frame True {
          n245 = Array Max & Min(array=w548) -> (max value=w542:dbl, min value=w540:dbl)  [unwired: 2 out]
          n246 = Array Size(array=w548) -> (size(s)=w543:i32)
          n247 = Subtract(x=w542, y=w540) -> (x-y=w544:dbl)
          n248 = Divide(x=w544, y=w543) -> (x/y=w541:dbl)
          n249 = control-ref of="Curve fit"() -> (w546:refnum<vi>)
          n250 = control-ref of="Fit deviation"() -> (w545:refnum<vi>)
          n251 = property on="Property Node" class="WFGraph (strict)"(reference=w546, "XScale.NameLbl.Text"=w547, "XScale.Maximum"=w542, "XScale.Minimum"=w540) -> ()  [unwired: 1 in, 2 out]
          n252 = property on="Property Node" class="WFGraph (strict)"(reference=w545, "XScale.NameLbl.Text"=w547, "XScale.Maximum"=w542, "XScale.Minimum"=w540, "XScale.Offset"=w540, "XScale.Multiplier"=w541) -> ()  [unwired: 1 in, 2 out]
        }
      }
      n253 = call "Convert to Dynamic Data12"("Array"=w533) -> ("Dynamic Data Type"=w518:dynamicdata)  [unwired: 3 in]
      n254 = Build Array(w531, w532) -> (→"Curve fit":dbl[][])
      n255 = Subtract(x=w531, y=w532) -> (x-y=w513:dbl[])
      n256 = call "Build Table3"("Signals"=w518) -> ("Table"=w517:string[][])  [unwired: 4 in, 6 out]
      n257 = Multiply(x=w513, y=100) -> (x*y=→"Fit deviation":dbl[])
      n258 = call <vilib>:"Correlation Coefficient.vi"("Y"=w532, "X"=w531) -> ("r^2"=→"R^2":dbl, "correlation coefficient r"=→"Correlation\ncoefficient (R)":dbl)  [unwired: 8 in]
      n259 = Transpose 2D Array(2D array=w517) -> (transposed array=→"Coefficients":string[][])
    }
  }
